vi "Yokogawa - rename waveform.vi"(10 "Numeric":i32, 11 "Waveform in":waveform(dbl)) -> (3 "Waveform out":waveform(dbl))   [LabVIEW 2013]
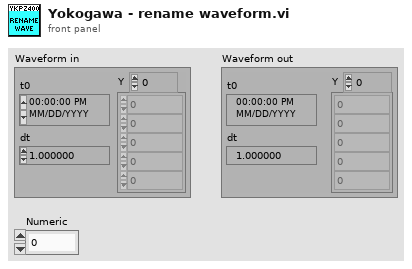
[diagram p1: front panel]
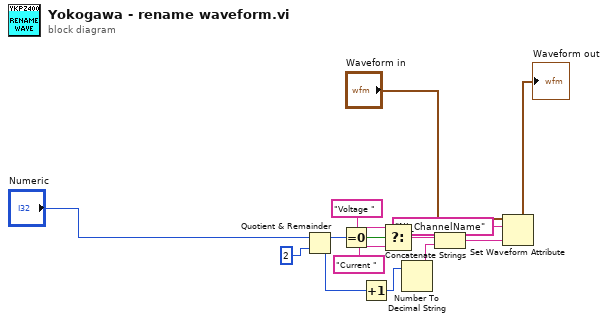
[diagram p0: block diagram]
diagram:
  n1 = Quotient & Remainder(x="Numeric", y=2) -> (x-y*floor(x/y)=w5:i32, floor(x/y)=w14:i32)
  n2 = Equal To 0?(x=w5) -> (x = 0?=w6:bool)
  n3 = Increment(x=w14) -> (x+1=w12:i32)
  n4 = Select(t="Voltage ", s=w6, f="Current ") -> (s? t:f=w9:string)
  n5 = Number To Decimal String(number=w12) -> (decimal integer string=w10:string)  [unwired: 1 in]
  n6 = Concatenate Strings(w9, w10) -> (w11:string)
  n7 = Set Waveform Attribute(5:w11, 6:"NI_ChannelName" ("name"), 7:"Waveform in") -> (3:→"Waveform out":waveform(dbl))  [unwired: 1 in, 2 out]
